vi "Next_Field.vi"(7 "Field and Temp Array Controller":cluster{"Field (T)":dbl[], "Temps (K)":dbl[]}, 8 "error in (no error)":errorcluster, 9 "MagQ In":refnum<queue>, 10 "Temp and Field Range in":T2, 11 "Queue in":refnum<queue>) -> (0 "error out":errorcluster, 1 "MagQ Out":refnum<queue>, 2 "Temp and Field Range out":T2, 3 "Queue out":refnum<queue>, 5 "PSU Status Out":T1={"Ramp Target"=enum."ZERO", "Pause"=FALSE, "Switch Heater"=FALSE, "Persistent Field"=0.0, "Persistent Current"=0.0, "Tesla"=FALSE, "Output (T)"=0.0, "Output (A)"=0.0, "X Trip"=enum."DISABLED", "Ramp Rate (A/s)"=0.0, "V Limit (V)"=0.0, "Heater Voltage"=0.0, "MAX Setpoint (A)"=0.0, "MAX Setpoint (T)"=0.0, "MID Setpoint (A)"=0.0, "MID Setpoint (T)"=0.0, "Lock"=FALSE, "Field Constant"=0.0, "Remote"=FALSE, "Direction"=enum."POSITIVE", "Helium Level"=0, "Quench !"=FALSE, "Voltage"=0.0, "V Limit !"=FALSE, "Ramping"=FALSE, "At Target"=FALSE, "Trip Field"=0.0, "Trip Current"=0.0, "Current State"=enum."1. INIT MAG", "MAG Reference"="COM4"} {"Trip Current" format="%.3f"; "Trip Field" format="%.4f"; "Voltage" format="%.2f"; "Field Constant" format="%.6f"; "MID Setpoint (T)" format="%.4f"; "MID Setpoint (A)" format="%.3f"; "MAX Setpoint (T)" format="%.4f"; "MAX Setpoint (A)" format="%.3f"; "Heater Voltage" format="%.2f"; "V Limit (V)" format="%.2f"; "Ramp Rate (A/s)" format="%.3f"; "Output (A)" format="%.3f"; "Output (T)" format="%.4f"; "Persistent Current" format="%.3f"; "Persistent Field" format="%.4f"})   [LabVIEW 2025]
uses:
  CTLS/Sweeper.ctl
  CTLS/PSU Status.ctl
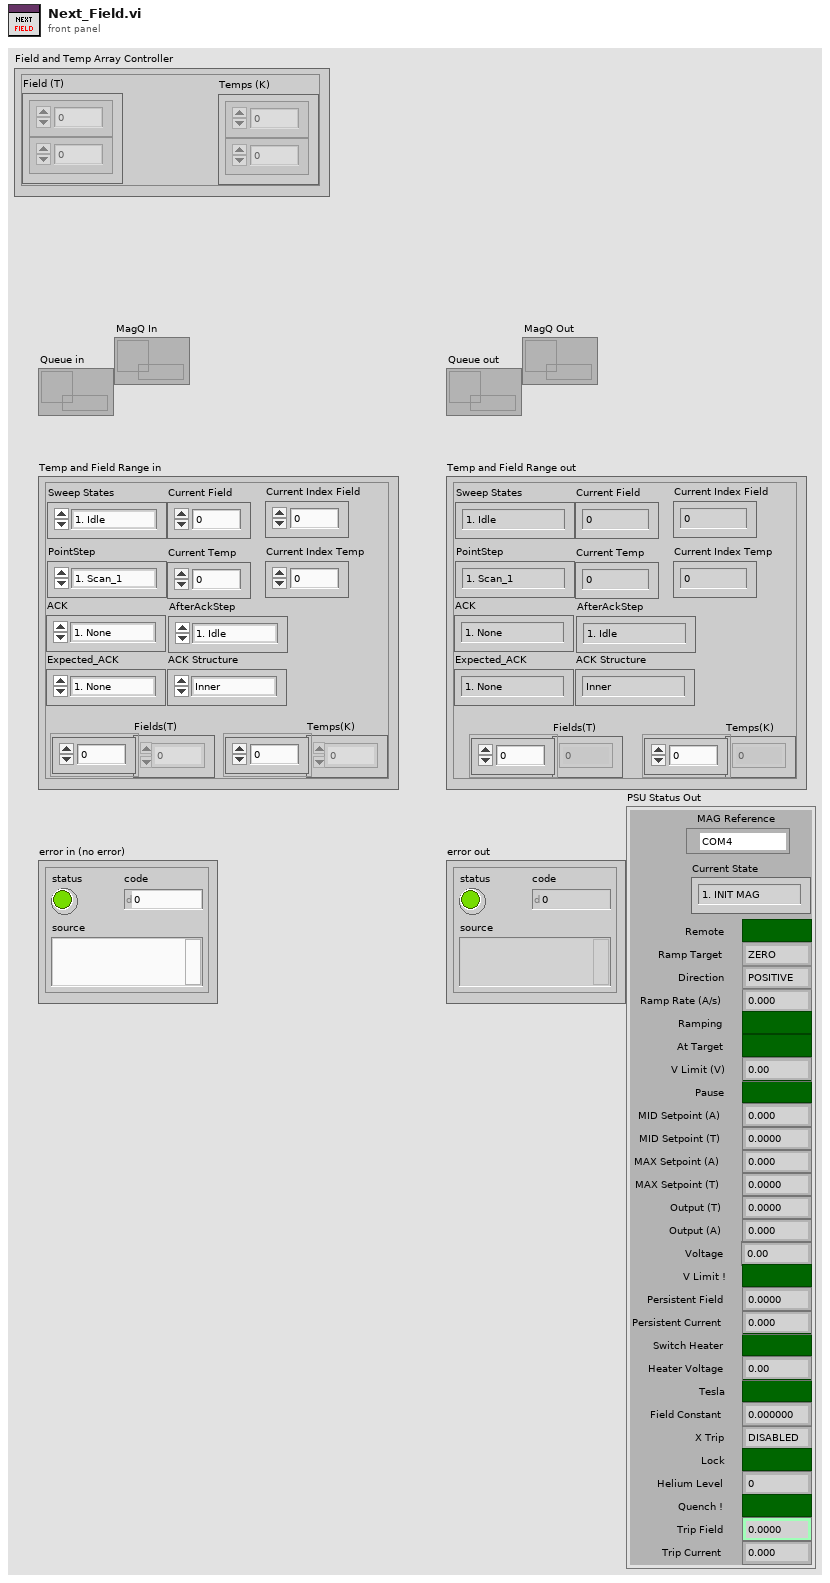
[diagram p1: front panel]
types:
  T1 = typedef "PSU Status.ctl" = cluster{"Ramp Target":enum16{"ZERO", "MID", "MAX"}, "Pause":bool, "Switch Heater":bool, "Persistent Field":dbl, "Persistent Current":dbl, "Tesla":bool, "Output (T)":dbl, "Output (A)":dbl, "X Trip":enum16{"DISABLED", "ENABLED", "ACTIVE"}, "Ramp Rate (A/s)":dbl, "V Limit (V)":dbl, "Heater Voltage":dbl, "MAX Setpoint (A)":dbl, "MAX Setpoint (T)":dbl, "MID Setpoint (A)":dbl, "MID Setpoint (T)":dbl, "Lock":bool, "Field Constant":dbl, "Remote":bool, "Direction":enum16{"POSITIVE", "NEGATIVE", "OPEN", "UNIPOLAR"}, "Helium Level":u16, "Quench !":bool, "Voltage":dbl, "V Limit !":bool, "Ramping":bool, "At Target":bool, "Trip Field":dbl, "Trip Current":dbl, "Current State":enum16{"1. INIT MAG", "2. MAG ON", "3. MAG_STAB", "4. MAG IDLE", "5. MAG OFF (Reset)"}, "MAG Reference":refnum<visa-resource-name>}
  T2 = typedef "Sweeper.ctl" = cluster{"Temps(K)":dbl[], "Fields(T)":dbl[], "Sweep States":enum16{"1. Idle", "2. Start", "3. Apply_Config", "4. Run_Point_Step", "5. Wait ACK", "6. Next Field", "7. Next Temp", "8. Stop"}, "PointStep":enum16{"1. Scan_1", "2. DC_SF_1", "3. DC_BS_1", "4. Bias", "5. Scan_2", "6. DC_SF_2", "7. DC_BS_2", "8. Done"}, "Current Field":dbl, "Current Temp":dbl, "Expected_ACK":enum16{"1. None", "2. TempStable", "3. FieldStable", "4. ConfigApplied", "5. ScanDone", "6. BiasDone", "7. DriftDone (SF)", "8. DrifDone (BS)", "9. Done"}, "ACK":enum16{"1. None", "2. TempStable", "3. FieldStable", "4. ConfigApplied", "5. ScanDone", "6. BiasDone", "7. DriftDone (SF)", "8. DrifDone (BS)", "9. Done"}, "AfterAckStep":enum16{"1. Idle", "2. Start", "3. Apply_Config", "4. Run_Point_Step", "5. Wait ACK", "6. Next Field", "7. Next Temp", "8. Stop"}, "Current Index Field":i32, "Current Index Temp":i32, "ACK Structure ":enum16{"Inner", "Outer"}}
  T3 = enum16{"1. Scan_1", "2. DC_SF_1", "3. DC_BS_1", "4. Bias", "5. Scan_2", "6. DC_SF_2", "7. DC_BS_2", "8. Done"}
  T4 = enum16{"1. Idle", "2. Start", "3. Apply_Config", "4. Run_Point_Step", "5. Wait ACK", "6. Next Field", "7. Next Temp", "8. Stop"}
  T5 = enum16{"1. None", "2. TempStable", "3. FieldStable", "4. ConfigApplied", "5. ScanDone", "6. BiasDone", "7. DriftDone (SF)", "8. DrifDone (BS)", "9. Done"}
  T6 = enum16{"1. INIT MAG", "2. MAG ON", "3. MAG_STAB", "4. MAG IDLE", "5. MAG OFF (Reset)"}
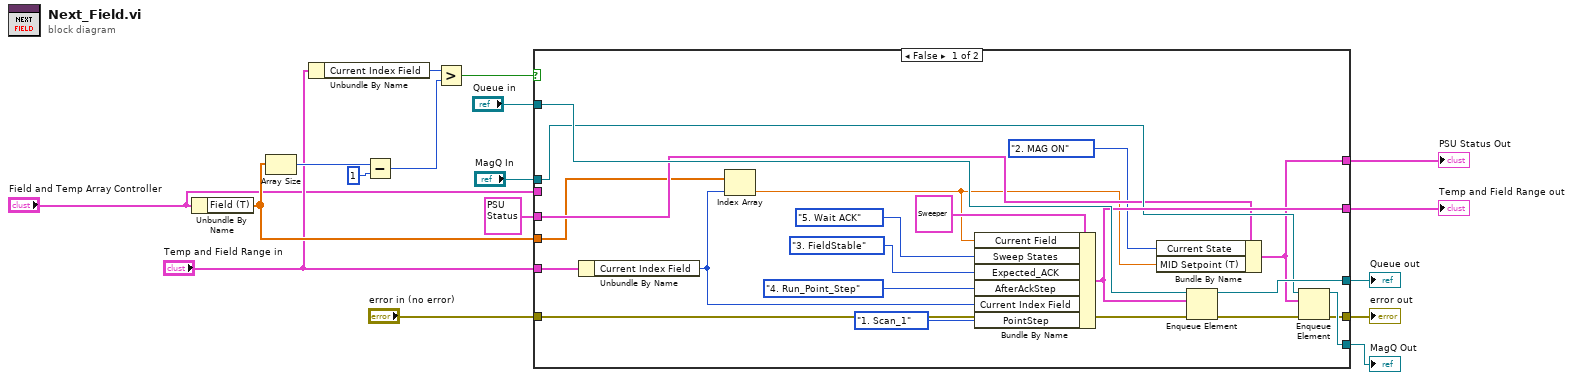
[diagram p0: block diagram]
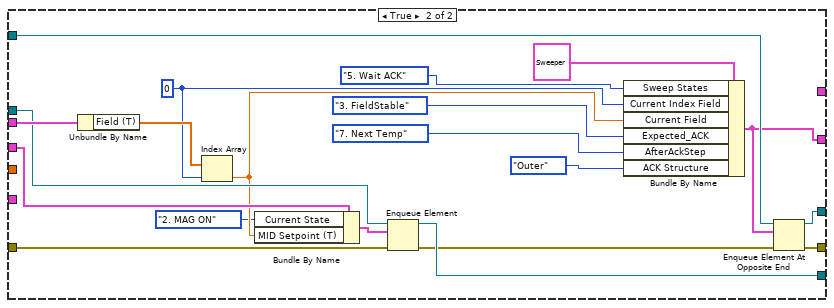
[diagram p2: hidden frame]
diagram:
  n1 = Unbundle By Name("Field and Temp Array Controller") -> ("Field (T)"=w3:dbl[])
  n2 = Array Size(array=w3) -> (size(s)=w10:i32)
  n3 = Unbundle By Name("Temp and Field Range in") -> ("Current Index Field"=w8:i32)
  n4 = Subtract(x=w10, y=1) -> (x-y=w11:i32)
  n5 = Greater?(x=w8, y=w11) -> (0:w9:bool)
  n6 = case shown="False" w9 {
    tunnel: [w33 w48] -> w13
    tunnel: "Queue in" -> [w37 w49]
    tunnel: [w35 w47] -> w15
    tunnel: [w25 w56] -> w16
    tunnel: "error in (no error)" -> [w36 w42]
    tunnel: "MagQ In" -> [w32 w44]
    tunnel: T1 {"Ramp Target"=enum."ZERO", "Pause"=FALSE, "Switch Heater"=FALSE, "Persistent Field"=0.0, "Persistent Current"=0.0, "Tesla"=FALSE, "Output (T)"=0.0, "Output (A)"=0.0, "X Trip"=enum."DISABLED", "Ramp Rate (A/s)"=0.0, "V Limit (V)"=0.0, "Heater Voltage"=0.0, "MAX Setpoint (A)"=0.0, "MAX Setpoint (T)"=0.0, "MID Setpoint (A)"=0.0, "MID Setpoint (T)"=0.0, "Lock"=FALSE, "Field Constant"=0.0, "Remote"=FALSE, "Direction"=enum."POSITIVE", "Helium Level"=0, "Quench !"=FALSE, "Voltage"=0.0, "V Limit !"=FALSE, "Ramping"=FALSE, "At Target"=FALSE, "Trip Field"=0.0, "Trip Current"=0.0, "Current State"=enum."1. INIT MAG", "MAG Reference"="COM4"} ("PSU Status In") -> [w29 w46]
    tunnel: [w31 w43] -> w6
    tunnel: [w26 _] -> w5
    tunnel: w3 -> [w24 _]
    tunnel: "Field and Temp Array Controller" -> [_ w54]
    tunnel: "Temp and Field Range in" -> [w23 _]
    frame False {
      n7 = Unbundle By Name(w23) -> ("Current Index Field"=w19:i32)
      n8 = Index Array(array=w24, index=w19) -> (element=w27:dbl)
      n9 = Bundle By Name(cluster=T2 {"Temps(K)"=[], "Fields(T)"=[], "Sweep States"=enum."1. Idle", "PointStep"=enum."1. Scan_1", "Current Field"=0.0, "Current Temp"=0.0, "Expected_ACK"=enum."1. None", "ACK"=enum."1. None", "AfterAckStep"=enum."1. Idle", "Current Index Field"=0, "Current Index Temp"=0, "ACK Structure "=enum."Inner"} ("Temp and Field Range"), "Current Field"=w27, "Sweep States"=T4."5. Wait ACK", "Expected_ACK"=T5."3. FieldStable", "AfterAckStep"=T4."4. Run_Point_Step", "Current Index Field"=w19, "PointStep"=T3."1. Scan_1") -> (w33:T2)
      n10 = Bundle By Name(cluster=w29, "Current State"=T6."2. MAG ON", "MID Setpoint (T)"=w27) -> (w26:T1)
      n11 = Enqueue Element(queue=w37, element=w33, error in (no error)=w36) -> (queue out=w35:refnum<queue>, error out=w30:errorcluster)  [unwired: 1 in, 1 out]
      n12 = Enqueue Element(queue=w32, element=w26, error in (no error)=w30) -> (queue out=w31:refnum<queue>, error out=w25:errorcluster)  [unwired: 1 in, 1 out]
    }
    frame True {
      w50 = 0 ("Current Index Field")
      n13 = Unbundle By Name(w54) -> ("Field (T)"=w55:dbl[])
      n14 = Index Array(array=w55, index=w50) -> (element=w40:dbl)
      n15 = Bundle By Name(cluster=w46, "Current State"=T6."2. MAG ON", "MID Setpoint (T)"=w40) -> (w45:T1)
      n16 = Enqueue Element(queue=w44, element=w45, error in (no error)=w42) -> (queue out=w43:refnum<queue>, error out=w41:errorcluster)  [unwired: 1 in, 1 out]
      n17 = Bundle By Name(cluster=T2 {"Temps(K)"=[], "Fields(T)"=[], "Sweep States"=enum."1. Idle", "PointStep"=enum."1. Scan_1", "Current Field"=0.0, "Current Temp"=0.0, "Expected_ACK"=enum."1. None", "ACK"=enum."1. None", "AfterAckStep"=enum."1. Idle", "Current Index Field"=0, "Current Index Temp"=0, "ACK Structure "=enum."Inner"} ("Temp and Field Range"), "Sweep States"=T4."5. Wait ACK", "Current Index Field"=w50, "Current Field"=w40, "Expected_ACK"=T5."3. FieldStable", "AfterAckStep"=T4."7. Next Temp", "ACK Structure"=enum16{"Inner", "Outer"}."Outer") -> (w48:T2)
      n18 = Enqueue Element At Opposite End(queue=w49, element=w48, error in (no error)=w41) -> (queue out=w47:refnum<queue>, error out=w56:errorcluster)  [unwired: 1 in, 1 out]
    }
  }
  "error out" <- w16
  "Queue out" <- w15
  "Temp and Field Range out" <- w13
  "MagQ Out" <- w6
  "PSU Status Out" <- w5
